vi "convert_to_16bit.vi"(1 "Floating point":sgl) -> (0 "Output Array":u16[](array[numeric]))   [LabVIEW 2011]
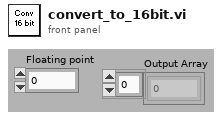
[diagram p1: front panel]
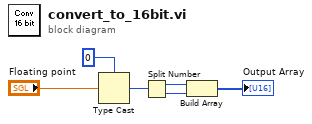
[diagram p0: block diagram]
diagram:
  n1 = Type Cast(type=u32 0, x="Floating point") -> (*(type *) &x=w4:u32)
  n2 = Split Number(x=w4) -> (hi(x)=w3:u16, lo(x)=w2:u16)
  n3 = Build Array(w3, w2) -> (→"Output Array":u16[])
